vi "DeleteFirstRow(SubVI).vi"(11 "TblParam in":sgl[][](array[numeric])) -> (3 "TblParam out":sgl[][](array[numeric]))   [LabVIEW 2017]
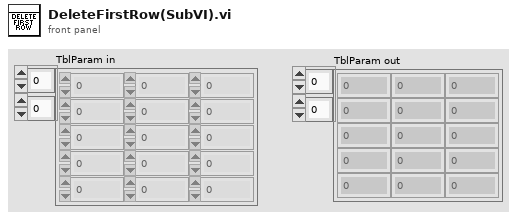
[diagram p1: front panel]
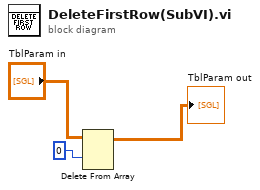
[diagram p0: block diagram]
diagram:
  n1 = Delete From Array(array="TblParam in", index (row)=0) -> (array with subset deleted=→"TblParam out":sgl[][])  [unwired: 2 in, 1 out]
